vi "DumbDash Find Control Names.vi"(11 "Controls":refnum<vi>[](array[refnum])) -> (3 "Dashboard Names":string[](array[string]))   [LabVIEW 2015]
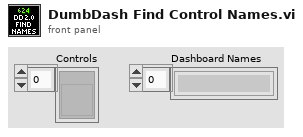
[diagram p1: front panel]
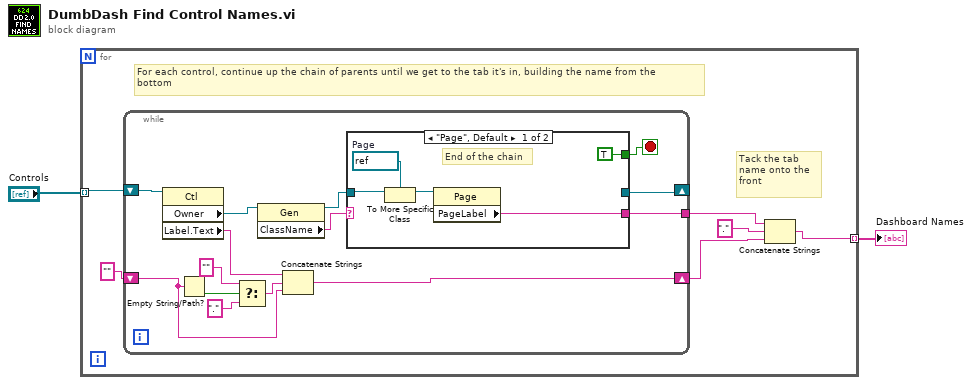
[diagram p0: block diagram]
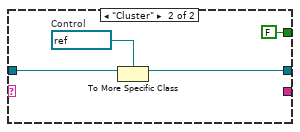
[diagram p2: hidden frame]
diagram:
  n1 = for {
    tunnel: "Controls" -> [w8] mode=indexing
    tunnel: [w4] -> w1 mode=indexing
    # "Tack the tab\nname onto the \nfront"
    # "For each control, continue up the chain of parents until we get to the tab it's in, building the name from the\nbottom"
    n2 = while {
      shift-right: [w11] -> _
      shift-left: w8 -> [w21]
      shift-right: [w19] -> w5
      shift-left: "" ("Label.Text") -> [w14]
      tunnel: [w9] -> w6
      stop <- w10 stop-if-true
      n3 = property class="Ctl"(reference=w21) -> ("Owner"=w22:refnum<vi>, "Label.Text"=w20:string)  [unwired: 1 in, 2 out]
      n4 = Empty String/Path?(string/path=w14) -> (empty?=w18:bool)
      n5 = Select(t="" ("Label.Text"), s=w18, f=".") -> (s? t:f=w15:string)
      n6 = property class="Gen"(reference=w22) -> (reference out=w12:refnum<vi>, "ClassName"=w13:string)  [unwired: 1 in, 1 out]
      n7 = Concatenate Strings(w20, w15, w14) -> (w19:string)
      n8 = case shown="\"Page\", Default" w13 {
        tunnel: w12 -> [w26 w31]
        tunnel: [_ w29] -> w11
        tunnel: [TRUE FALSE] -> w10
        tunnel: [w23 _] -> w9
        frame "Page", Default {
          w25 = refnum<vi> refnum  # Page
          # "End of the chain"
          n9 = To More Specific Class(target class=w25, reference=w26) -> (specific class reference=w24:refnum<vi>)  [unwired: 1 in, 1 out]
          n10 = property class="Page"(reference=w24) -> ("PageLabel"=w23:string)  [unwired: 1 in, 2 out]
        }
        frame "Cluster" {
          w30 = refnum<vi> refnum  # Control
          n11 = To More Specific Class(target class=w30, reference=w31) -> (specific class reference=w29:refnum<vi>)  [unwired: 1 in, 1 out]
        }
      }
    }
    n12 = Concatenate Strings(w6, "." ("string"), w5) -> (w4:string)
  }
  "Dashboard Names" <- w1
